vi "Status Read Error.vi"(8 "error in (no error)":errorcluster, 11 "Status Reference":T1) -> (0 "error out":errorcluster, 1 "Error":i32, 3 "Status Reference out":T1)   [LabVIEW 2021, in "Status.lvlib"]
uses:
  Status.lvlib
  Ctl/control.ctl
  Ctl/State.ctl
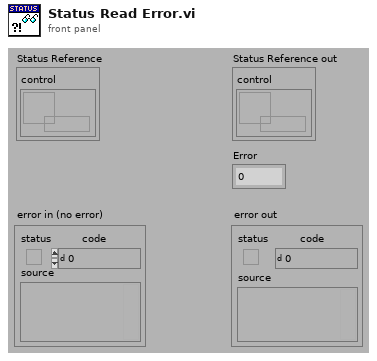
[diagram p1: front panel]
types:
  T1 = typedef "Status.lvlib/control.ctl" = cluster{"control":refnum<data-value>}
  T2 = typedef "Status.lvlib/State.ctl" = enum8{"initialization", "redefine", "standby", "connect", "wait to reconnect", "wait to reset timeout", "configure", "requests", "close connection", "stop"}
  T3 = cluster{"set_state":cluster{"Start":bool, "WrEn":bool, "Stop":bool}, "state":cluster{"errors":i32, "connect":bool, "state":T2}}
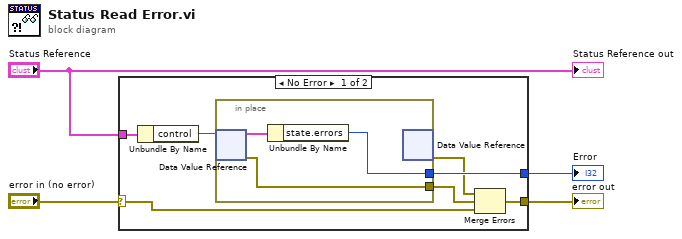
[diagram p0: block diagram]
diagram:
  n1 = case shown="No Error" "error in (no error)" {
    selector: "error in (no error)" -> [w5 w15]
    tunnel: [w9 w15] -> w1
    tunnel: [w11 _] -> w2
    tunnel: "Status Reference" -> [w10 _]
    frame No Error {
      n2 = Unbundle By Name(w10) -> ("control"=w6:refnum<data-value>)
      n3 = in-place {
        in-place-border: [w12] -> w11
        in-place-border: [w14] -> w7
        n4 = in-place-dvr #1(w6) -> (w13:T3, w14:errorcluster)
        n5 = Unbundle By Name(w13) -> ("state.errors"=w12:i32)
        n6 = in-place-dvr #1() -> (w8:errorcluster)  [unwired: 1 in, 1 out]
      }
      n7 = Merge Errors(w8, w7, w5) -> (w9:errorcluster)
    }
    frame Error {
    }
  }
  "error out" <- w1
  "Error" <- w2
  "Status Reference out" <- "Status Reference"
